vi "Result Check.vi"(0 "Lower":dbl, 1 "Upper":dbl, 2 "Test Data":dbl, 5 "Unit":string) -> (6 "Result":bool, 7 "Result String Array Out":string[](array[string]))   [LabVIEW 2018]
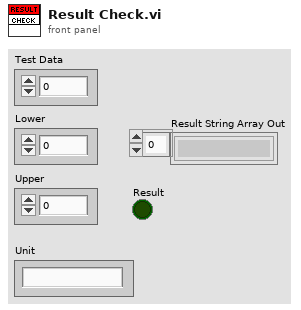
[diagram p1: front panel]
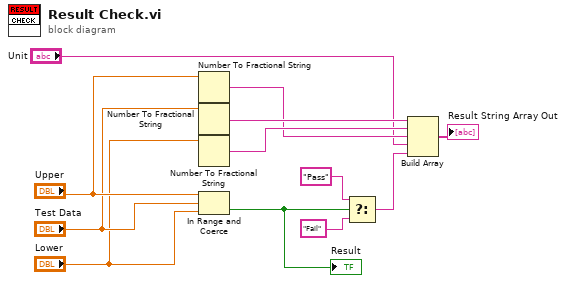
[diagram p0: block diagram]
diagram:
  n1 = Number To Fractional String(number="Upper") -> (F-format string=w7:string)  [unwired: 3 in]
  n2 = Number To Fractional String(number="Test Data") -> (F-format string=w9:string)  [unwired: 3 in]
  n3 = Number To Fractional String(number="Lower") -> (F-format string=w8:string)  [unwired: 3 in]
  n4 = In Range and Coerce(upper limit="Upper", x="Test Data", lower limit="Lower") -> (In Range?=w6:bool)  [unwired: 1 out]
  "Result" <- w6
  n5 = Select(t="Pass", s=w6, f="Fail") -> (s? t:f=w1:string)
  n6 = Build Array(w9, w8, w7, "Unit", w1) -> (→"Result String Array Out":string[])
